vi "Control PAS Heater.vi"(0 "Session Handle in":T1, 7 "Start?":bool, 11 "error in (no error)":errorcluster) -> (4 "Session Handle out":T1, 6 "Success?":bool, 8 "Error Code":string, 15 "error out":errorcluster)   [LabVIEW 2015, in "PAS.lvclass"]
uses:
  PAS.lvclass
  Typedefs/Session Handle.ctl
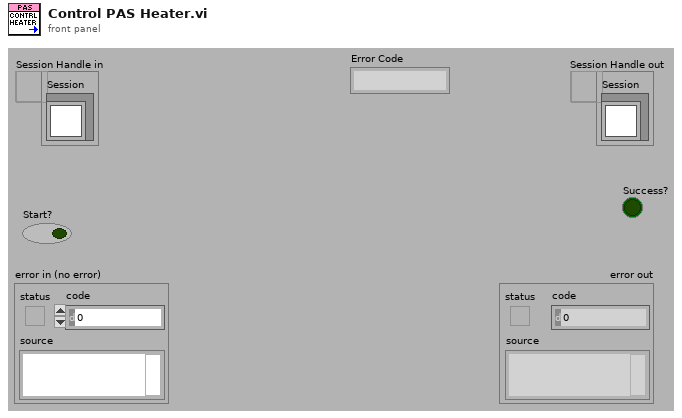
[diagram p1: front panel]
types:
  T1 = typedef "PAS.lvclass/Session Handle.ctl" = refnum<data-value>
  T2 = typedef "XNET Frame CAN.ctl" = cluster{"timestamp":timestamp, "payload":u8[], "identifier":u32, "type":T3, "extended?":bool, "echo?":bool}
  T3 = typedef "XNET Frame Type CAN.ctl" = u8
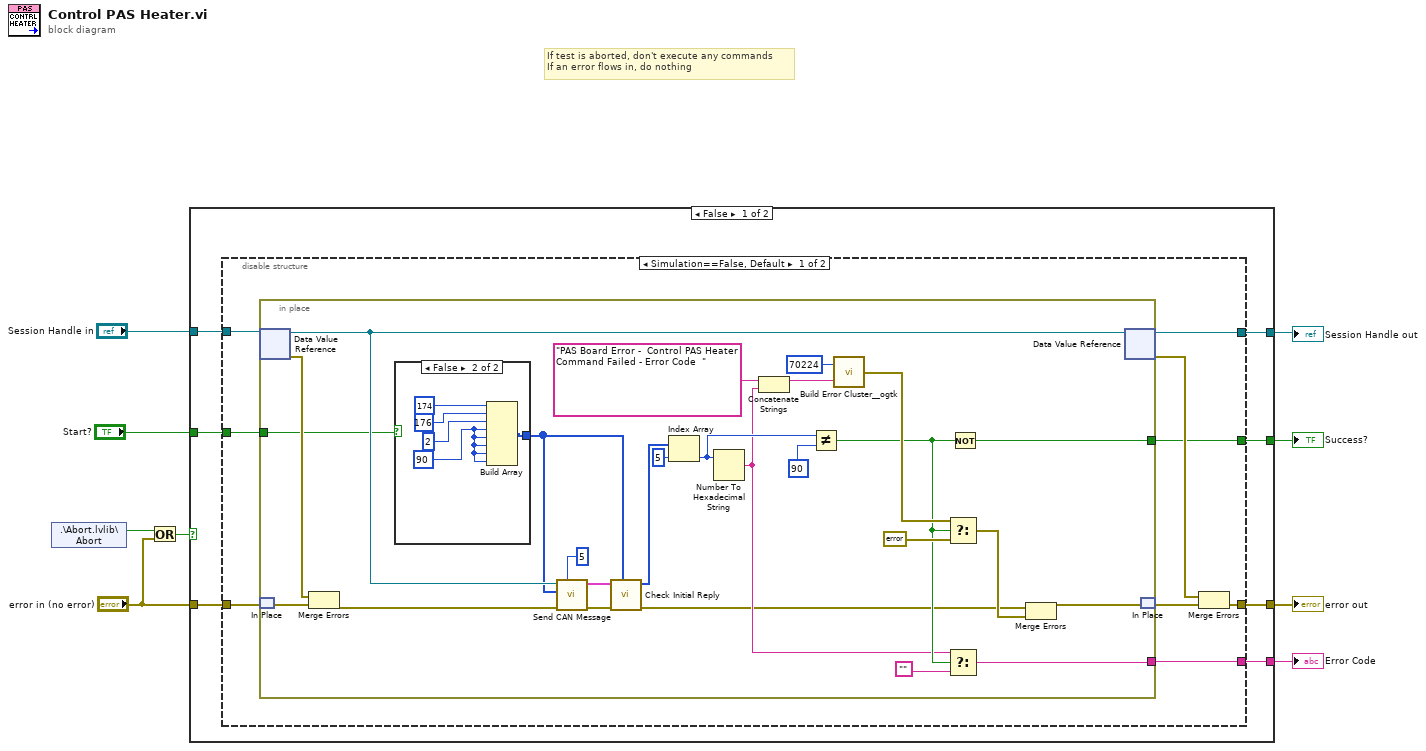
[diagram p0: block diagram]
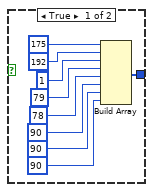
[diagram p2: hidden frame]
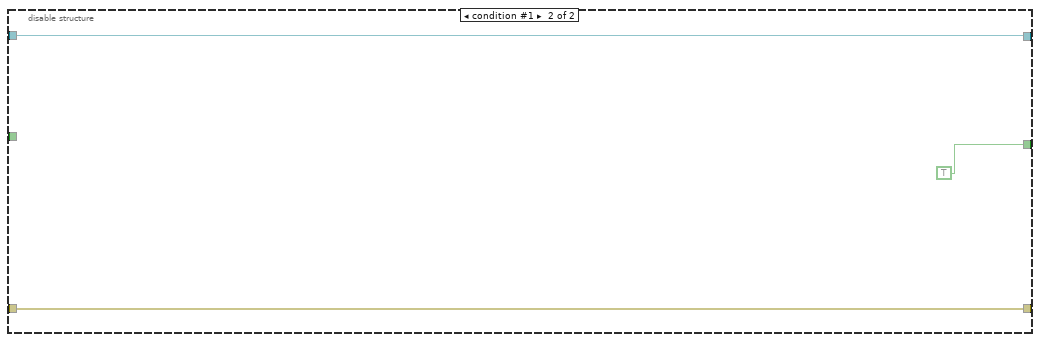
[diagram p3: hidden frame]
diagram:
  # "If test is aborted, don't execute any commands\nIf an error flows in, do nothing"
  n1 = shared-variable ".\\Abort.lvlib\\Abort"() -> (w6:bool)  [unwired: 1 in, 1 out]
  n2 = Or(x=w6, y="error in (no error)") -> (x .or. y?=w4:bool)
  n3 = case shown="False" w4 {
    tunnel: [w16 w70] -> w8
    tunnel: [w15 w69] -> w7
    tunnel: "Session Handle in" -> [w14 w70]
    tunnel: "error in (no error)" -> [w13 w69]
    tunnel: [w12 _] -> w3
    tunnel: "Start?" -> [w11 _]
    tunnel: [w10 _] -> w1
    frame False {
      n4 = disable-structure shown="Simulation==False, Default" {
        disable-tunnel: [w25 w68] -> w16
        disable-tunnel: [w22 w67] -> w15
        disable-tunnel: w14 -> [w21 w68]
        disable-tunnel: w13 -> [w20 w67]
        disable-tunnel: [w19 TRUE] -> w12
        disable-tunnel: w11 -> [w18 _]
        disable-tunnel: [w17 _] -> w10
        frame condition #0 (active) {
          n5 = in-place {
            in-place-border: [w41] -> w19
            in-place-border: w18 -> [w40]
            in-place-border: [w28] -> w17
            n6 = in-place-dvr #1(w21) -> (w47:refnum<class "PAS.lvclass">, w50:errorcluster)
            n7 = in-place-match #2(w20) -> (w49:errorcluster)
            n8 = Merge Errors(w50, w49) -> (w48:errorcluster)
            n9 = case shown="False" w40 {
              tunnel: [w56 w63] -> w39
              frame True {
                n10 = Build Array(u8 175 ("new element/subarray"), u8 192 ("new element/subarray"), u8 1 ("new element/subarray"), u8 79 ("new element/subarray"), u8 78 ("new element/subarray"), u8 90 ("new element/subarray"), u8 90 ("new element/subarray"), u8 90 ("new element/subarray")) -> (w56:u8[])
              }
              frame False {
                w61 = u8 90 ("new element/subarray")
                n11 = Build Array(u8 174 ("new element/subarray"), u8 176 ("new element/subarray"), u8 2 ("new element/subarray"), w61, w61, w61, w61, w61) -> (w63:u8[])
              }
            }
            n12 = call "Send CAN Message.vi"("Number of Retries"=5, "error in (no error)"=w48, "payload"=w39, "Gas In"=w47) -> ("error out"=w27:errorcluster, "Reply"=w45:T2[])  [unwired: 5 in, 1 out]
            n13 = call "Check Initial Reply.vi"("Write Message"=w39, "error in (no error)"=w27, "Reply"=w45) -> ("error out"=w26:errorcluster, "Data Packet"=w38:u8[])  [unwired: 5 in, 2 out]
            n14 = Index Array(array=w38, index=5) -> (element=w34:u8)
            n15 = Number To Hexadecimal String(2:w34) -> (0:w29:string)  [unwired: 1 in]
            n16 = Concatenate Strings("PAS Board Error -  Control PAS Heater Command Failed - Error Code  " ("string"), w29) -> (w35:string)
            n17 = Not Equal?(x=w34, y=u8 90 ("new element/subarray")) -> (x != y?=w30:bool)
            n18 = call <userlib>:"Build Error Cluster__ogtk.vi"("String to Prepend to source (\"\")"=w35, "code"=70224) -> ("error out"=w43:errorcluster)
            n19 = Select(t=w43, s=w30, f=errorcluster {"status"=FALSE, "code"=0, "source"=""}) -> (s? t:f=w32:errorcluster)
            n20 = Select(t=w29, s=w30, f="") -> (s? t:f=w28:string)
            n21 = Not(x=w30) -> (.not. x?=w41:bool)
            n22 = Merge Errors(w26, w32) -> (w51:errorcluster)
            n23 = in-place-dvr #1(w47) -> (w25:T1, w23:errorcluster)
            n24 = in-place-match #2(w51) -> (w24:errorcluster)
          }
          n25 = Merge Errors(w23, w24) -> (w22:errorcluster)
        }
        frame condition #1 {
        }
      }
    }
    frame True {
    }
  }
  "Session Handle out" <- w8
  "error out" <- w7
  "Success?" <- w3
  "Error Code" <- w1
